vi "Init.vi"(10 "Iterate":i32) -> (3 "Iterate Msg Strategy out":refnum<class "Iterate Msg Strategy.lvclass">)   [LabVIEW 2021, in "Hello World Event.lvlib" / "Iterate Msg Strategy.lvlib" / "Iterate Msg Strategy.lvclass"]
uses:
  Iterate Msg Strategy.lvclass
  Iterate Msg Strategy.lvclass/Iterate Msg Strategy.ctl
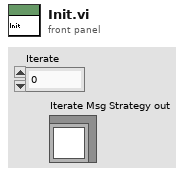
[diagram p1: front panel]
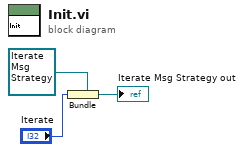
[diagram p0: block diagram]
diagram:
  n1 = Bundle "Bundle"(cluster=refnum<class "Iterate Msg Strategy.lvclass"> refnum ("TEMPLATE Msg Strategy out"), "Iterate") -> (→"Iterate Msg Strategy out":refnum<class "Iterate Msg Strategy.lvclass">)
